vi "calculator.vi"() -> ()   [LabVIEW 2016]
panel:
  in  ".":bool
  out "Result":string
  in  "stop":bool
  in  "2":bool
  in  "C":bool
  in  "=":bool
  in  "\\":bool
  in  "*":bool
  in  "-":bool
  in  "+":bool
  in  "9":bool
  in  "8":bool
  in  "5":bool
  # "Bing's calculator"
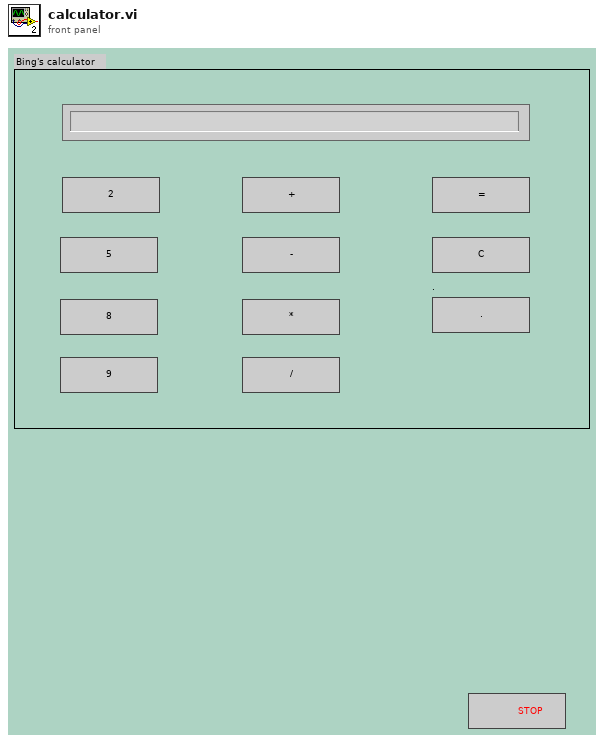
[diagram p1: front panel]
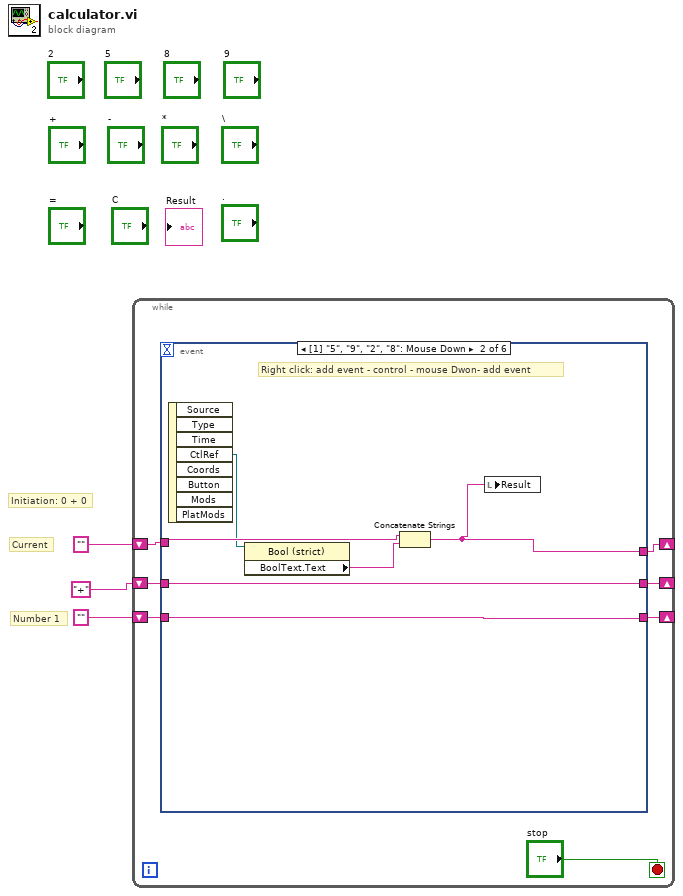
[diagram p0: block diagram]
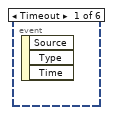
[diagram p2: hidden frame]
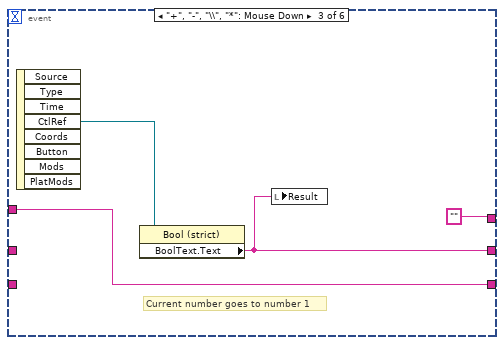
[diagram p3: hidden frame]
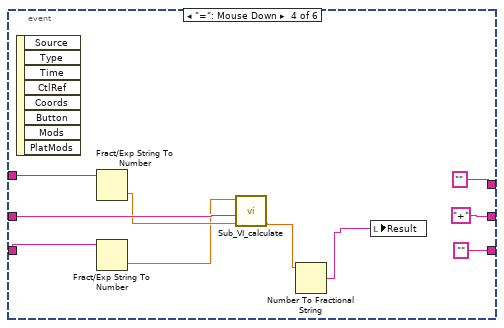
[diagram p4: hidden frame]
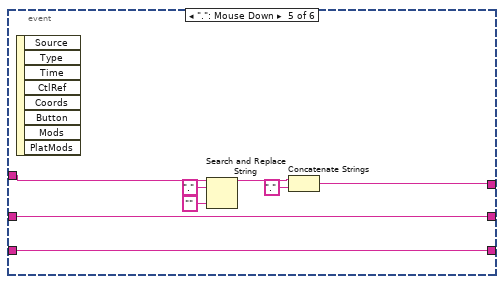
[diagram p5: hidden frame]
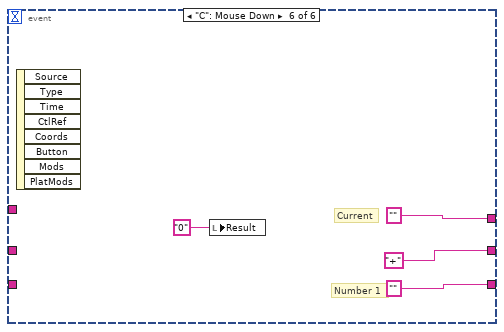
[diagram p6: hidden frame]
diagram:
  # "Initiation: 0 + 0"
  # "Number 1"
  # "Current"
  n1 = while {
    shift-right: [w6] -> _
    shift-left: "" -> [w9]
    shift-right: [w4] -> _
    shift-left: "+" -> [w8]
    shift-right: [w5] -> _
    shift-left: "" -> [w7]
    stop <- "stop" stop-if-true
    n2 = event shown="[1] \"5\", \"9\", \"2\", \"8\": Mouse Down" {
      selector: _ -> [_ _ _ _ _ _]
      dyn-events: _ -> [_ _ _ _ _ _]
      timeout: _ -> [_ _ _ _ _ _]
      tunnel: w9 -> [_ w16 w20 w30 w36 _]
      tunnel: w8 -> [_ w13 _ w29 w37 _]
      tunnel: w7 -> [_ w14 _ w28 w38 _]
      tunnel: [_ w12 "" "" w31 ""] -> w6
      tunnel: [_ w14 w20 "" w38 ""] -> w5
      tunnel: [_ w13 w18 "+" w37 "+"] -> w4
      event Timeout {
        n3 = event-data() -> ()  [unwired: 1 in, 3 out]
      }
      event "5", "9", "2", "8": Mouse Down {
        # "Right click: add event - control - mouse Dwon- add event"
        n4 = event-data() -> ("CtlRef"=w11:refnum<vi>)  [unwired: 1 in, 7 out]
        n5 = property class="Bool (strict)"(reference=w11) -> ("BoolText.Text"=w15:string)  [unwired: 1 in, 2 out]
        n6 = Concatenate Strings(w16, w15) -> (w12:string)
        n7 = local write "Result"(w12) -> ()
      }
      event "+", "-", "\\", "*": Mouse Down {
        # "Current number goes to number 1"
        n8 = event-data() -> ("CtlRef"=w17:refnum<vi>)  [unwired: 1 in, 7 out]
        n9 = property class="Bool (strict)"(reference=w17) -> ("BoolText.Text"=w18:string)  [unwired: 1 in, 2 out]
        n10 = local write "Result"(w18) -> ()
      }
      event "=": Mouse Down {
        n11 = event-data() -> ()  [unwired: 1 in, 8 out]
        n12 = Fract/Exp String To Number(string=w30) -> (number=w25:dbl)  [unwired: 3 in, 1 out]
        n13 = Fract/Exp String To Number(string=w28) -> (number=w24:dbl)  [unwired: 3 in, 1 out]
        n14 = call "Sub_VI_calculate.vi"("Num 2"=w25, "Combo Box"=w29, "Num 1"=w24) -> ("Result"=w22:dbl)  [unwired: 8 in]
        n15 = Number To Fractional String(number=w22) -> (F-format string=w21:string)  [unwired: 3 in]
        n16 = local write "Result"(w21) -> ()
      }
      event ".": Mouse Down {
        n17 = event-data() -> ()  [unwired: 1 in, 8 out]
        n18 = Search and Replace String(input string=w36, search string=".", replace string="" ("replace string (\"\")")) -> (result string=w33:string)  [unwired: 5 in, 3 out]
        n19 = Concatenate Strings(w33, "." ("string")) -> (w31:string)
      }
      event "C": Mouse Down {
        # "Number 1"
        # "Current"
        n20 = event-data() -> ()  [unwired: 1 in, 8 out]
        n21 = local write "Result"("0") -> ()
      }
    }
  }
